vi "Encode ClientID.vi"(10 "Client ID (empty: generate new)":string) -> (2 "valid Client ID":bool, 3 "Length-Prefixed Field":u8[](array[numeric]) format="%08b")   [LabVIEW 2013, in "MQTT_Control_Packets.lvlib" / "ControlPacket.lvclass"]
uses:
  ControlPacket.lvclass
panel:
  out "Array":i16[](array[numeric])
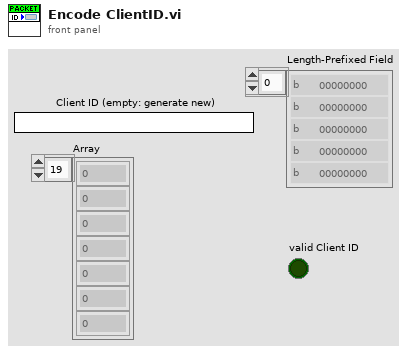
[diagram p1: front panel]
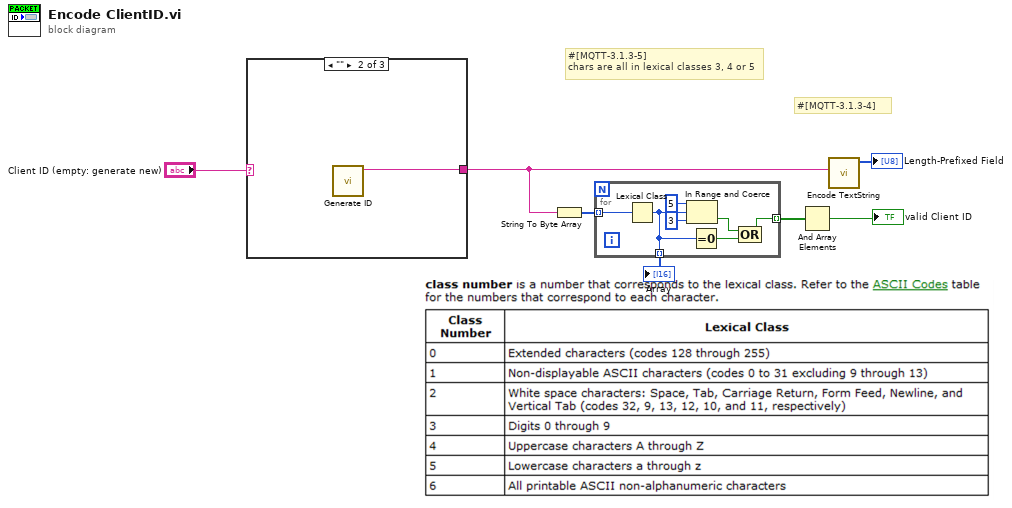
[diagram p0: block diagram]
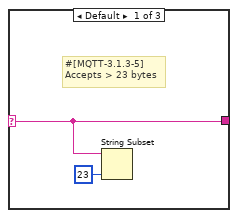
[diagram p2: hidden frame]
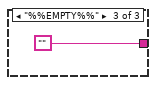
[diagram p3: hidden frame]
diagram:
  # "#[MQTT-3.1.3-5]\nchars are all in lexical classes 3, 4 or 5"
  # "#[MQTT-3.1.3-4]"
  n1 = case shown="\"\"" "Client ID (empty: generate new)" {
    selector: "Client ID (empty: generate new)" -> [w8 _ _]
    tunnel: [w8 w10 ""] -> w6
    frame Default {
      # "#[MQTT-3.1.3-5]\nAccepts > 23 bytes"
      n2 = String Subset(string=w8, length (rest)=23 ("length (rest)")) -> ()  [unwired: 1 in, 1 out]
    }
    frame "" {
      n3 = call "Generate ID.vi"() -> ("ID"=w10:string)  [unwired: 11 in]
    }
    frame "%%EMPTY%%" {
    }
  }
  n4 = String To Byte Array(string=w6) -> (unsigned byte array=w3:u8[])
  n5 = for {
    tunnel: w3 -> [w18] mode=indexing
    tunnel: [w12] -> w5 mode=indexing
    tunnel: [w14] -> w1 mode=indexing
    n6 = Lexical Class(1:w18) -> (0:w14:i16)
    n7 = In Range and Coerce(upper limit=i16 5, x=w14, lower limit=i16 3) -> (In Range?=w13:bool)  [unwired: 1 out]
    n8 = Equal To 0?(x=w14) -> (x = 0?=w15:bool)
    n9 = Compound Arithmetic op=OR(w13, w15) -> (w12:bool)
  }
  "Array" <- w1
  n10 = And Array Elements(Boolean array=w5) -> (logical AND=→"valid Client ID":bool)
  n11 = call "Encode TextString.vi"("Text String"=w6) -> ("Length-Prefixed Field"=→"Length-Prefixed Field":u8[])  [unwired: 10 in]
